vi "Parse Response JSON.vi"(8 "error in (no error)":errorcluster, 10 "Response JSON":string, 11 "RGetInputKindList in":refnum<class "RGetInputKindList.lvclass">) -> (0 "error out":errorcluster, 3 "RGetInputKindList out":refnum<class "RGetInputKindList.lvclass">)   [LabVIEW 2022 SP3, in "obs-websocket-lv.lvlib" / "RGetInputKindList.lvclass"]
uses:
  RGetInputKindList.lvclass
  RGetInputKindList.lvclass/RGetInputKindList.ctl
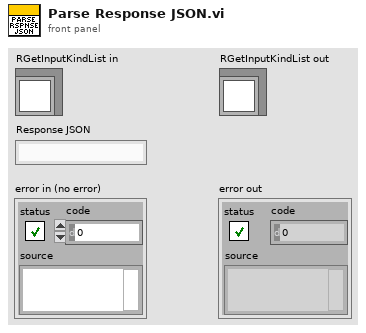
[diagram p1: front panel]
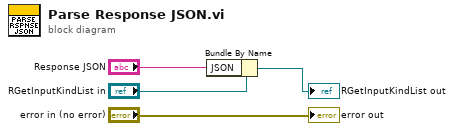
[diagram p0: block diagram]
diagram:
  n1 = Bundle By Name(cluster="RGetInputKindList in", "JSON"="Response JSON") -> (→"RGetInputKindList out":refnum<class "RGetInputKindList.lvclass">)
  "error out" <- "error in (no error)"
